vi "Write Class Data for Manager SubPanel.vi"(8 "error in (no error)":errorcluster, 10 "Class Data for Manager SubPanel":T1, 11 "CIF_Manager_UI in":refnum<class "CIF_Manager_UI.lvclass">) -> (0 "error out":errorcluster, 3 "CIF_Manager_UI out":refnum<class "CIF_Manager_UI.lvclass">)   [LabVIEW 2021, in "CIF_Manager_UI.lvclass"]
uses:
  CIF_Manager_UI.lvclass
  C:/Program Files/National Instruments/LabVIEW 2021/vi.lib/CIF Foundation/CIF Core/CIFUI/CIF_UI.lvclass
  Typedef/Class Data for Manager SubPanel.ctl
  <vilib>/CIF Foundation/CIF Core/CIFUI/Typedef/Class Data for SubPanel.ctl
  <vilib>/CIF Foundation/CIF Core/CIFUI/Typedef/Core UI References.ctl
  <vilib>/CIF Foundation/CIF Core/CIFUI/Typedef/Run Listen Button.ctl
  <vilib>/CIF Foundation/CIF Core/CIFUI/Typedef/SubPanel Events.ctl
  <vilib>/CIF Foundation/CIF Core/CIFUI/Typedef/New Connection Plugin Event Data.ctl
  Typedef/Core Manager UI References.ctl
  Typedef/Channel Connection.ctl
  Typedef/New Plugin.ctl
  Typedef/CIF_Manager_UI_Tab.ctl
  CIFPluginManager/typedef/New Connection Event Data.ctl
  <vilib>/gRPC/LabVIEW gRPC Library/Shared/grpcId.ctl
  CIF_Manager_UI.lvclass/CIF_Manager_UI.ctl
  <vilib>/CIF Foundation/CIF Core/CIFUI/CIF_UI.lvclass/CIF_UI.ctl
  <vilib>/CIF Foundation/CIF Core/CIFUI/CIF_UI.lvclass
  D:/dev/CIF_Manager/src/CIFPluginManager/UI/CIFManagerUI Class/CIF_Manager_UI.lvclass
  <vilib>/gRPC/LabVIEW gRPC Library/grpc-lvsupport-release.lvlib
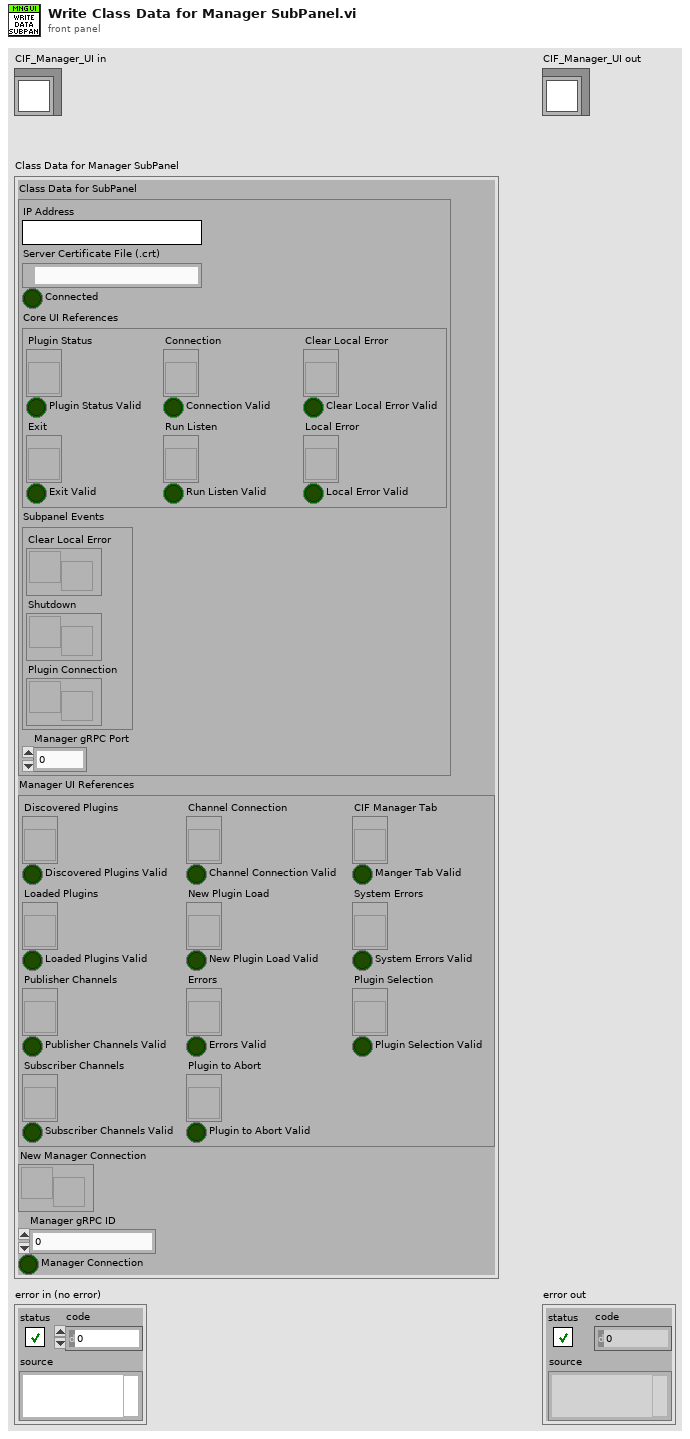
[diagram p1: front panel]
types:
  T1 = typedef "CIF_Manager_UI.lvclass/Class Data for Manager SubPanel.ctl" = cluster{"Class Data for SubPanel":T2, "Manager UI References":T5, "New Manager Connection":refnum<user-event>, "Manager gRPC ID":T6, "Manager Connection":bool}
  T2 = typedef "CIF_UI.lvclass/Class Data for SubPanel.ctl" = cluster{"IP Address":string, "Server Certificate File (.crt)":path, "Connected":bool, "Core UI References":T3, "Subpanel Events":T4, "Manager gRPC Port":u16}
  T3 = typedef "CIF_UI.lvclass/Core UI References.ctl" = cluster{"Plugin Status":refnum<vi>, "Plugin Status Valid":bool, "Connection":refnum<vi>, "Connection Valid":bool, "Exit":refnum<vi>, "Exit Valid":bool, "Run Listen":refnum<vi>, "Run Listen Valid":bool, "Clear Local Error":refnum<vi>, "Clear Local Error Valid":bool, "Local Error":refnum<vi>, "Local Error Valid":bool}
  T4 = typedef "CIF_UI.lvclass/SubPanel Events.ctl" = cluster{"Clear Local Error":refnum<user-event>, "Shutdown":refnum<user-event>, "Plugin Connection":refnum<user-event>}
  T5 = typedef "CIF_Manager_UI.lvclass/Core Manager UI References.ctl" = cluster{"Discovered Plugins":refnum<vi>, "Discovered Plugins Valid":bool, "Loaded Plugins":refnum<vi>, "Loaded Plugins Valid":bool, "Publisher Channels":refnum<vi>, "Publisher Channels Valid":bool, "Subscriber Channels":refnum<vi>, "Subscriber Channels Valid":bool, "Channel Connection":refnum<vi>, "Channel Connection Valid":bool, "New Plugin Load":refnum<vi>, "New Plugin Load Valid":bool, "Errors":refnum<vi>, "Errors Valid":bool, "Plugin to Abort":refnum<vi>, "Plugin to Abort Valid":bool, "CIF Manager Tab":refnum<vi>, "Manger Tab Valid":bool, "System Errors":refnum<vi>, "System Errors Valid":bool, "Plugin Selection":refnum<vi>, "Plugin Selection Valid":bool}
  T6 = typedef "grpc-lvsupport-release.lvlib/grpcId.ctl" = u64
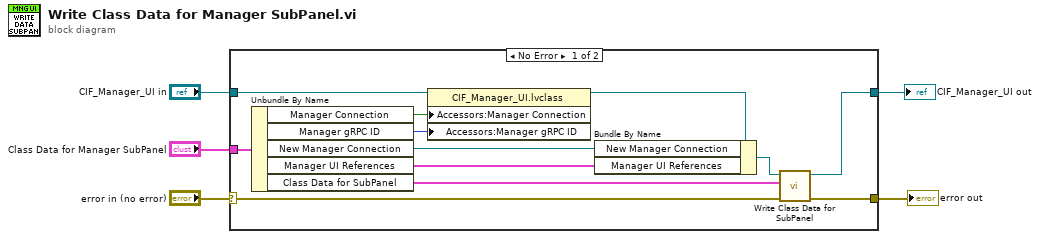
[diagram p0: block diagram]
diagram:
  n1 = case shown="No Error" "error in (no error)" {
    selector: "error in (no error)" -> [w15 w19]
    tunnel: [w11 w19] -> w4
    tunnel: [w12 w18] -> w2
    tunnel: "CIF_Manager_UI in" -> [w9 w18]
    tunnel: "Class Data for Manager SubPanel" -> [w17 _]
    frame No Error {
      n2 = Unbundle By Name(w17) -> ("Manager Connection"=w7:bool, "Manager gRPC ID"=w8:T6, "New Manager Connection"=w10:refnum<user-event>, "Manager UI References"=w14:T5, "Class Data for SubPanel"=w16:T2)
      n3 = property class="CIF_Manager_UI.lvclass"(reference=w9, "Accessors:Manager Connection"=w7, "Accessors:Manager gRPC ID"=w8) -> (reference out=w6:refnum<class "CIF_Manager_UI.lvclass">)  [unwired: 1 in, 1 out]
      n4 = Bundle By Name(cluster=w6, "New Manager Connection"=w10, "Manager UI References"=w14) -> (w13:refnum<class "CIF_Manager_UI.lvclass">)
      n5 = call <vilib>:"Write Class Data for SubPanel.vi"("error in (no error)"=w15, "Class Data for SubPanel"=w16, "CIF_UI in"=w13) -> ("error out"=w11:errorcluster, "CIF_UI in"=w12:refnum<class "CIF_Manager_UI.lvclass">)  [unwired: 7 in]
    }
    frame Error {
    }
  }
  "error out" <- w4
  "CIF_Manager_UI out" <- w2
